vi "fgv_cmd.vi"(7 "Mode":T1=enum."Update", 8 "error in":errorcluster, 10 "Value":string, 11 "System Log":refnum<vi>) -> (0 "error out":errorcluster)   [LabVIEW 2019]
uses:
  SubVIs/common/_ctrl/system-status.ctl
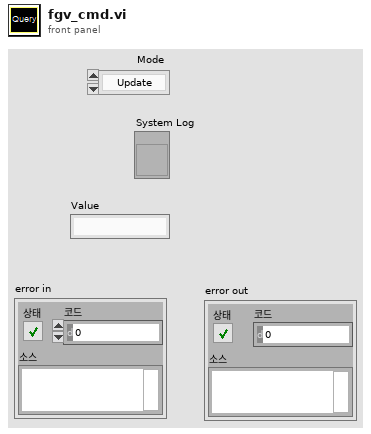
[diagram p1: front panel]
types:
  T1 = typedef "system-status.ctl" = enum16{"Initial", "Update", "Clear", "Read"}
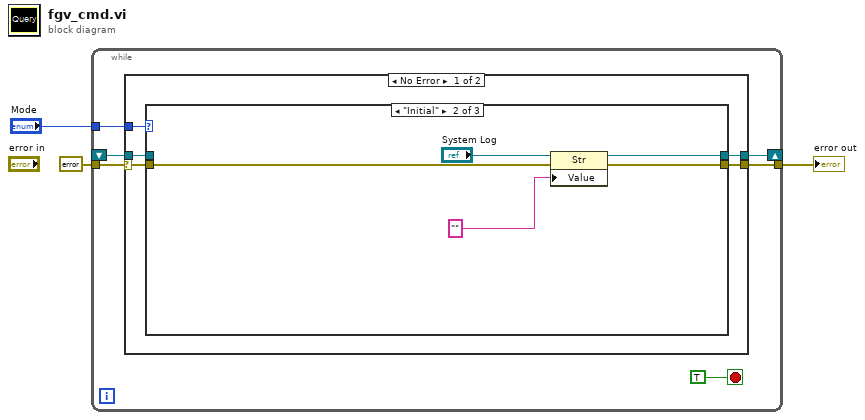
[diagram p0: block diagram]
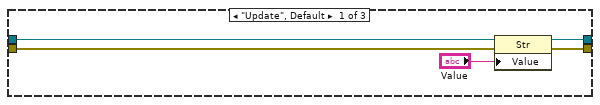
[diagram p2: hidden frame]
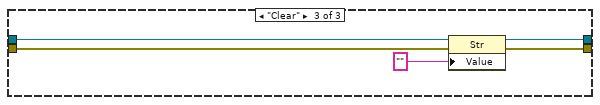
[diagram p3: hidden frame]
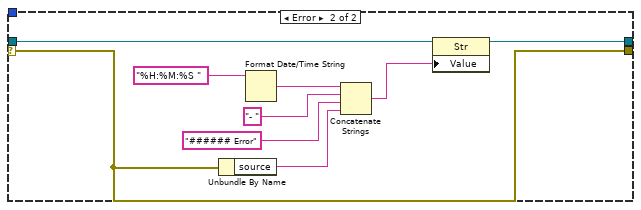
[diagram p4: hidden frame]
diagram:
  n1 = while {
    tunnel: errorcluster {"status"=FALSE, "code"=0, "source"=""} ("error in") -> [w4]
    tunnel: [w9] -> w3
    tunnel: "Mode" -> [w7]
    shift-right: [w6] -> _
    shift-left: _ -> [w5]
    stop <- TRUE stop-if-true
    n2 = case shown="No Error" w4 {
      selector: w4 -> [w10 w30]
      tunnel: [w14 w30] -> w9
      tunnel: w7 -> [w13 _]
      tunnel: [w12 w37] -> w6
      tunnel: w5 -> [w11 w38]
      frame No Error {
        n3 = case shown="\"Initial\"" w13 {
          tunnel: w11 -> [w17 _ w27]
          tunnel: w10 -> [w16 w21 w29]
          tunnel: [w19 w22 w28] -> w14
          tunnel: [w18 w23 w26] -> w12
          frame "Update", Default {
            n4 = property class="Str"(reference=w17, error in=w16, "Value"="Value") -> (reference out=w18:refnum<vi>, error out=w19:errorcluster)
          }
          frame "Initial" {
            n5 = property class="Str"(reference="System Log", error in=w21, "Value"="" ("값")) -> (reference out=w23:refnum<vi>, error out=w22:errorcluster)
          }
          frame "Clear" {
            n6 = property class="Str"(reference=w27, error in=w29, "Value"="" ("값")) -> (reference out=w26:refnum<vi>, error out=w28:errorcluster)
          }
        }
      }
      frame Error {
        n7 = Unbundle By Name(w30) -> ("source"=w32:string)
        n8 = Format Date/Time String(time format string (%c)="%H:%M:%S " ("시간 포맷 문자열 (%c)")) -> (date/time string=w35:string)  [unwired: 2 in]
        n9 = Concatenate Strings(w35, "- " ("포맷 문자열"), "###### Error" ("문자열"), w32) -> (w33:string)
        n10 = property class="Str"(reference=w38, "Value"=w33) -> (reference out=w37:refnum<vi>)  [unwired: 1 in, 1 out]
      }
    }
  }
  "error out" <- w3
